vi "System Options.vi"(8 "error in (no error)":errorcluster, 9 "Beeper (T: ON)":bool=TRUE, 10 "Display (T: ON)":bool=TRUE, 11 "VISA resource name":refnum<visa-resource-name>) -> (0 "error out":errorcluster, 3 "VISA resource name out":refnum<visa-resource-name>)   [LabVIEW 2020, in "Agilent 34405.lvlib"]
doc: "Allows users to turn off the instrument's beeper and display."
uses:
  <instrlib>/Agilent 34405/Agilent 34405.lvlib
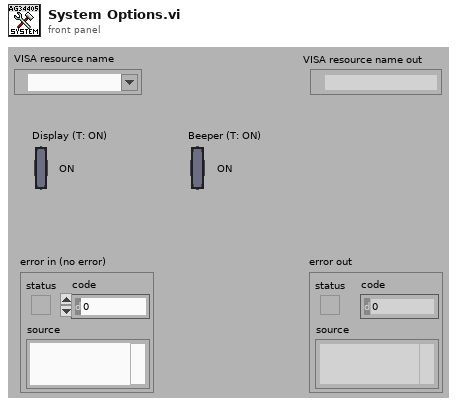
[diagram p1: front panel]
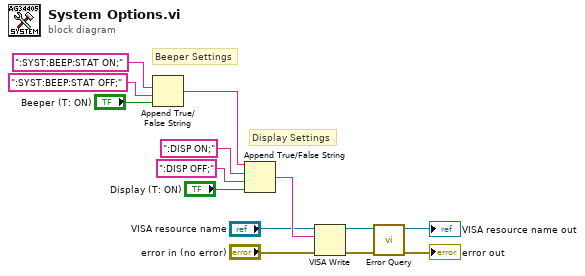
[diagram p0: block diagram]
diagram:
  # "Display Settings"
  # "Beeper Settings"
  n1 = Append True/False String(1:"Beeper (T: ON)", 2:":SYST:BEEP:STAT OFF;", 3:":SYST:BEEP:STAT ON;") -> (0:w1:string)  [unwired: 1 out]
  n2 = Append True/False String(1:"Display (T: ON)", 2:":DISP OFF;", 3:":DISP ON;", 4:w1) -> (0:w8:string)
  n3 = VISA Write(VISA resource name="VISA resource name", write buffer=w8, error in (no error)="error in (no error)") -> (VISA resource name out=w5:refnum<visa-resource-name>, error out=w4:errorcluster)  [unwired: 1 out]
  n4 = call <instrlib>:"Error Query.vi"("error in (no error)"=w4, "VISA resource name"=w5) -> ("error out"=→"error out":errorcluster, "VISA resource name out"=→"VISA resource name out":refnum<visa-resource-name>)  [unwired: 8 out]
